vi "Begin.vi"() -> (0 "error out":errorcluster)   [LabVIEW 2013]
uses:
  <vilib>/ActorFramework/Message Enqueuer/Message Enqueuer.lvclass
  Virtual Systems/Driver/Driver-Virtual/Driver-Virtual.lvclass
  Virtual Systems/Drive Train/Drive Train Class/Drive Train.lvclass
  <vilib>/ActorFramework/Message Queue/Message Queue.lvclass/Message Queue.ctl
  Robot Global.vi
  <vilib>/ActorFramework/Actor/Actor.lvclass
  <vilib>/ActorFramework/Message Queue/Message Queue.lvclass
panel:
  out "Caller-To-Actor Enqueuer":refnum<class "Message Enqueuer.lvclass">
  out "error out 2":errorcluster
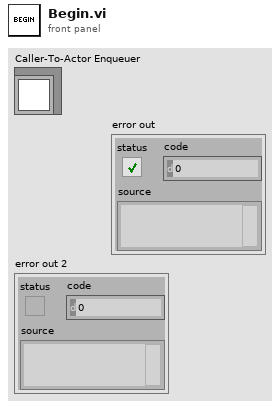
[diagram p1: front panel]
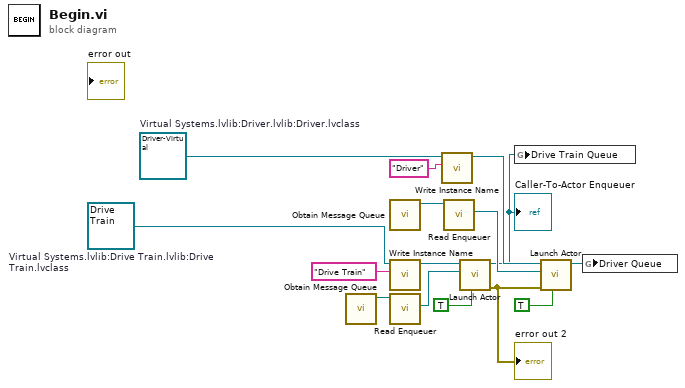
[diagram p0: block diagram]
diagram:
  w2 = refnum<class "Drive Train.lvclass"> refnum  # Virtual Systems.lvlib:Drive Train.lvlib:Drive Train.lvclass
  w12 = refnum<class "Driver-Virtual.lvclass"> refnum  # Virtual Systems.lvlib:Driver.lvlib:Driver.lvclass
  n1 = call <vilib>:"Obtain Message Queue.vi"() -> ("Message Queue"=w4:refnum<class "Message Queue.lvclass">)  [unwired: 10 in, 1 out]
  n2 = call <vilib>:"Obtain Message Queue.vi"() -> ("Message Queue"=w15:refnum<class "Message Queue.lvclass">)  [unwired: 10 in, 1 out]
  n3 = call-dynamic "Write Instance Name.vi"("Instance Name"="Drive Train", "System Actor in"=w2) -> ("System Actor out"=w7:refnum<class "Drive Train.lvclass">)  [unwired: 8 in, 1 out]
  n4 = call <vilib>:"Read Enqueuer.vi"("Message Queue"=w4) -> ("Message Enqueuer"=w5:refnum<class "Message Enqueuer.lvclass">)  [unwired: 10 in]
  n5 = call-dynamic "Write Instance Name.vi"("Instance Name"="Driver", "System Actor in"=w12) -> ("System Actor out"=w11:refnum<class "Driver-Virtual.lvclass">)  [unwired: 8 in, 1 out]
  n6 = call <vilib>:"Read Enqueuer.vi"("Message Queue"=w15) -> ("Message Enqueuer"=w14:refnum<class "Message Enqueuer.lvclass">)  [unwired: 10 in]
  n7 = call <vilib>:"Launch Actor.vi"("Open Actor Core front panel? (F)"=TRUE, "Actor-to-Caller Enqueuer"=w5, "Actor"=w7) -> ("error out"=w1:errorcluster, "Caller-To-Actor Enqueuer"=w3:refnum<class "Message Enqueuer.lvclass">)  [unwired: 7 in]
  "error out 2" <- w1
  "Caller-To-Actor Enqueuer" <- w3
  n8 = global write "Robot Global.vi" "Drive Train Queue"(w3) -> ()
  n9 = call <vilib>:"Launch Actor.vi"("Open Actor Core front panel? (F)"=TRUE, "error in (no error)"=w1, "Actor-to-Caller Enqueuer"=w14, "Actor"=w11) -> ("Caller-To-Actor Enqueuer"=w13:refnum<class "Message Enqueuer.lvclass">)  [unwired: 6 in, 1 out]
  n10 = global write "Robot Global.vi" "Driver Queue"(w13) -> ()
